vi "Check Path.vi"(8 "Error In":errorcluster, 10 "SAVE TYPE":u16(ring) items=["TDMS", "CSV"], 11 "file in":path) -> (0 "Error Out":errorcluster, 3 "path":path)   [LabVIEW 2025, in "Automotive Ethernet Bus Monitor UI.lvlib"]
uses:
  Automotive Ethernet Bus Monitor UI.lvlib
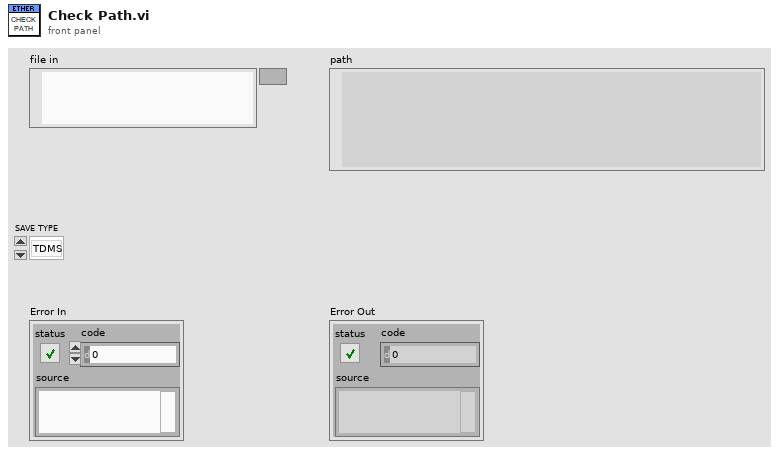
[diagram p1: front panel]
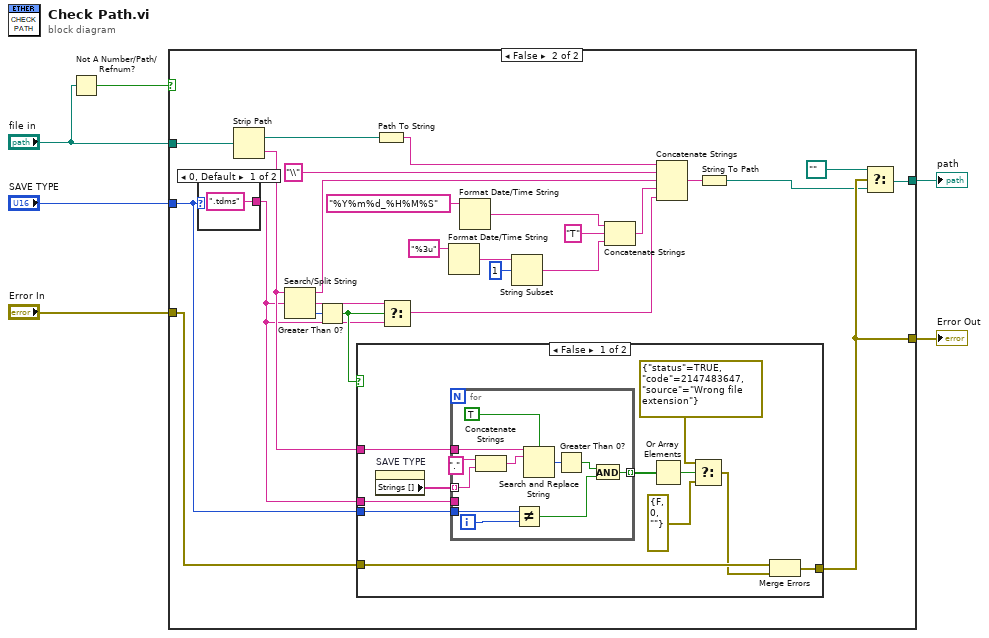
[diagram p0: block diagram]
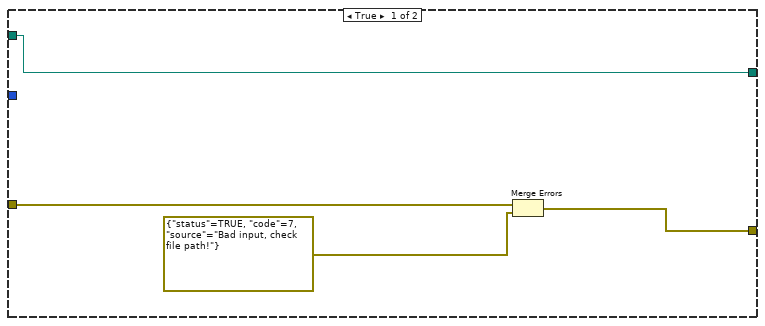
[diagram p2: hidden frame]
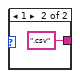
[diagram p4: hidden frame]
diagram:
  n1 = Not A Number/Path/Refnum?(number/path/refnum="file in") -> (NaN/Path/Refnum?=w6:bool)
  n2 = case shown="False" w6 {
    tunnel: [w9 w14] -> w3
    tunnel: [w7 w13] -> w1
    tunnel: "SAVE TYPE" -> [_ w15]
    tunnel: "file in" -> [w9 w20]
    tunnel: "Error In" -> [w8 w16]
    frame True {
      n3 = Merge Errors(w8, errorcluster {"status"=TRUE, "code"=7, "source"="Bad input, check file path!"} ("error constant")) -> (w7:errorcluster)
    }
    frame False {
      n4 = case shown="0, Default" w15 {
        tunnel: [".tdms" ("search string/char (-)") ".csv" ("search string/char (-)")] -> w17
        frame 0, Default {
        }
        frame 1 {
        }
      }
      n5 = Strip Path(path=w20) -> (stripped path=w33:path, name=w18:string)
      n6 = Search/Split String(string=w18, search string/char (-)=w17) -> (substring before match=w36:string, match + rest of string=w30:string, offset of match=w31:i32)  [unwired: 1 in]
      n7 = Greater Than 0?(x=w31) -> (x > 0?=w19:bool)
      n8 = case shown="False" w19 {
        tunnel: w18 -> [w46 _]
        tunnel: w17 -> [w45 _]
        tunnel: w16 -> [w41 w59]
        tunnel: [w38 w59] -> w13
        tunnel: w15 -> [w37 _]
        frame False {
          n9 = property on="SAVE TYPE" class="Ring (strict)"() -> ("Strings []"=w47:string[])  [unwired: 2 in, 2 out]
          n10 = for {
            tunnel: w47 -> [w49] mode=indexing
            tunnel: w46 -> [w53]
            tunnel: w45 -> [_]
            tunnel: [w56] -> w44 mode=indexing
            tunnel: w37 -> [w54]
            i -> [w55]
            n11 = Concatenate Strings("." ("string"), w49) -> (w48:string)
            n12 = Not Equal?(x=w54, y=w55) -> (x != y?=w57:bool)
            n13 = Search and Replace String(case sensitive?=TRUE ("ignore case? (F)"), input string=w53, search string=w48) -> (number of replacements=w51:i32)  [unwired: 5 in, 3 out]
            n14 = Greater Than 0?(x=w51) -> (x > 0?=w58:bool)
            n15 = And(x=w58, y=w57) -> (x .and. y?=w56:bool)
          }
          n16 = Or Array Elements(Boolean array=w44) -> (logical OR=w43:bool)
          n17 = Select(t=errorcluster {"status"=TRUE, "code"=2147483647, "source"="Wrong file extension"} ("error constant"), s=w43, f=errorcluster {"status"=FALSE, "code"=0, "source"=""} ("error constant")) -> (s? t:f=w39:errorcluster)
          n18 = Merge Errors(w41, w39) -> (w38:errorcluster)
        }
        frame True {
        }
      }
      n19 = Path To String(path=w33) -> (string=w32:string)
      n20 = Select(t=w30, s=w19, f=w17) -> (s? t:f=w29:string)
      n21 = Format Date/Time String(time format string (%c)="%3u") -> (date/time string=w26:string)  [unwired: 2 in]
      n22 = Format Date/Time String(time format string (%c)="%Y%m%d_%H%M%S") -> (date/time string=w27:string)  [unwired: 2 in]
      n23 = String Subset(string=w26, offset (0)=1) -> (substring=w28:string)  [unwired: 1 in]
      n24 = Concatenate Strings(w27, "T" ("string"), w28) -> (w21:string)
      n25 = Concatenate Strings(w32, "\\" ("string"), w36, w21, w29) -> (w34:string)
      n26 = String To Path(string=w34) -> (path=w12:path)
      n27 = Select(t=path "", s=w13, f=w12) -> (s? t:f=w14:path)
    }
  }
  "path" <- w3
  "Error Out" <- w1
